vi "ICNC Write Parameter.vi"(7 "TimeOut":u32, 8 "error in (no error)":errorcluster caption="entrée d'erreur (pas d'erreur)", 9 "WaitCompletion":i32, 10 "ParameterValue":u32, 11 "ParameterID":u32) -> (0 "error out":errorcluster caption="sortie d'erreur", 3 "function return":u32)   [LabVIEW 2012, in "ICNC2.lvlib"]
doc: "DWORD ICNC_WriteParameter( DWORD ParameterID,\n DWORD ParameterValue,\n BOOL WaitCompletion=TRUE,\n DWORD TimeOut=1000);"
uses:
  <userlib>/ICNC/ICNC2.lvlib
  <userlib>/ICNC/ICNC2.dll
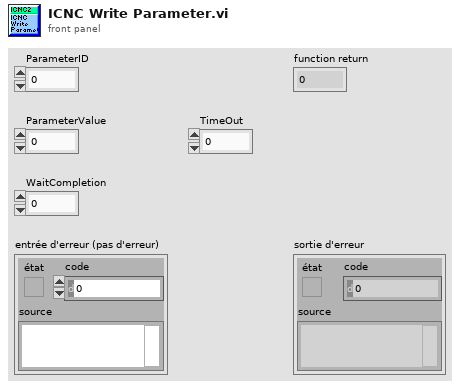
[diagram p1: front panel]
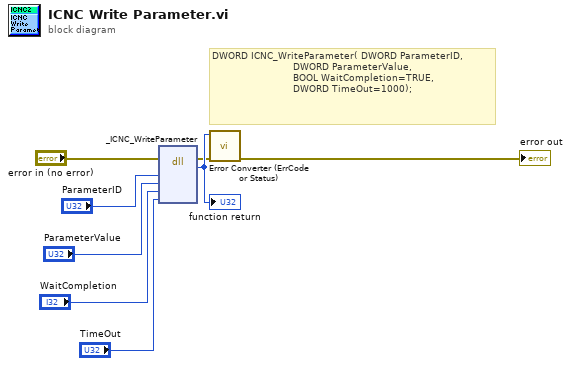
[diagram p0: block diagram]
diagram:
  # "DWORD ICNC_WriteParameter( DWORD ParameterID,\n                           DWORD ParameterValue,\n                           BOOL WaitCompletion=TRUE,\n                           DWORD TimeOut=1000);"
  n1 = dll-call lib="C:/Program Files (x86)/National Instruments/LabVIEW 2012/user.lib/ICNC/ICNC2.*" fn="_ICNC_WriteParameter"(error in="error in (no error)", "ParameterID"="ParameterID", "ParameterValue"="ParameterValue", "WaitCompletion"="WaitCompletion", "TimeOut"="TimeOut") -> (error out=w2:errorcluster, w8:u32)  [unwired: 6 in, 1 out]
  "function return" <- w8
  n2 = call <userlib>:"Error Converter (ErrCode or Status).vi"("error in (no error)"=w2, "error code"=w8) -> ("error out"=→"error out":errorcluster)  [unwired: 9 in]
